vi "DAE Simple Pendulum Simulation_Draw Coord.vi"(3 "picture in":picture) -> (1 "picture out":picture)   [LabVIEW 2023]
doc: "DAE Simple Pendulum Simulation Draw Coordinates"
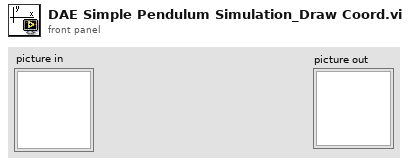
[diagram p1: front panel]
types:
  T1 = cluster{"horizontal":enum16{"left", "center", "right"}, "vertical":enum16{"top", "center", "bottom"}}
  T2 = cluster{"Font Name:":string, "Size":i16, "Strikeout?":bool, "Italic?":bool, "Underline?":bool, "Outline?":bool, "Shadow?":bool, "Bold?":bool}
  T3 = enum16{"User-specified Font", "Application Font", "System Font", "Dialog Font"}
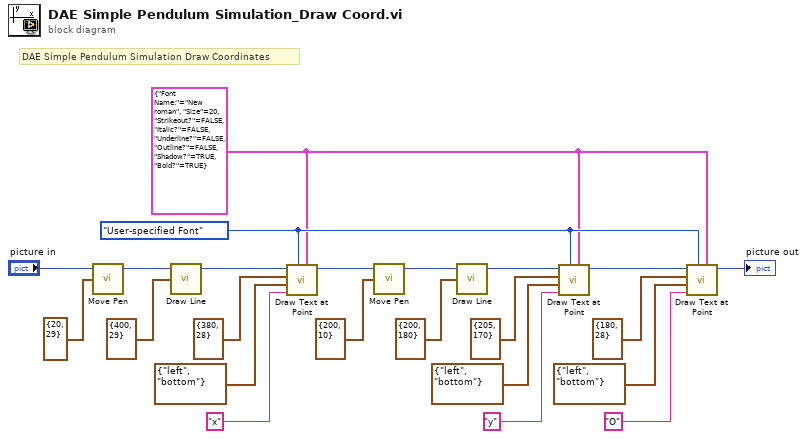
[diagram p0: block diagram]
diagram:
  w21 = T2 {"Font Name:"="New roman", "Size"=20, "Strikeout?"=FALSE, "Italic?"=FALSE, "Underline?"=FALSE, "Outline?"=FALSE, "Shadow?"=TRUE, "Bold?"=TRUE} ("[user-specified font]")
  w22 = T3."User-specified Font" ("desired font(Application)")
  # "DAE Simple Pendulum Simulation Draw Coordinates"
  n1 = call <vilib>:"Move Pen.vi"("new position"=cluster{"x":i16, "y":i16} {"x"=20, "y"=29}, "picture"="picture in") -> ("new picture"=w3:picture)  [unwired: 1 in, 2 out]
  n2 = call <vilib>:"Draw Line.vi"("picture"=w3, "end point"=cluster{"x":i16, "y":i16} {"x"=400, "y"=29}) -> ("new picture"=w5:picture)  [unwired: 3 in, 4 out]
  n3 = call <vilib>:"Draw Text at Point.vi"("[user-specified font]"=w21, "desired font(Application)"=w22, "text"="x", "alignment(left, top)"=T1 {"horizontal"=enum."left", "vertical"=enum."bottom"}, "origin"=cluster{"x":i16, "y":i16} {"x"=380, "y"=28}, "picture"=w5) -> ("new picture"=w9:picture)  [unwired: 3 in, 2 out]
  n4 = call <vilib>:"Move Pen.vi"("new position"=cluster{"x":i16, "y":i16} {"x"=200, "y"=10}, "picture"=w9) -> ("new picture"=w11:picture)  [unwired: 1 in, 2 out]
  n5 = call <vilib>:"Draw Line.vi"("picture"=w11, "end point"=cluster{"x":i16, "y":i16} {"x"=200, "y"=180}) -> ("new picture"=w13:picture)  [unwired: 3 in, 4 out]
  n6 = call <vilib>:"Draw Text at Point.vi"("[user-specified font]"=w21, "desired font(Application)"=w22, "text"="y", "alignment(left, top)"=T1 {"horizontal"=enum."left", "vertical"=enum."bottom"}, "origin"=cluster{"x":i16, "y":i16} {"x"=205, "y"=170}, "picture"=w13) -> ("new picture"=w17:picture)  [unwired: 3 in, 2 out]
  n7 = call <vilib>:"Draw Text at Point.vi"("[user-specified font]"=w21, "desired font(Application)"=w22, "text"="O", "alignment(left, top)"=T1 {"horizontal"=enum."left", "vertical"=enum."bottom"}, "origin"=cluster{"x":i16, "y":i16} {"x"=180, "y"=28}, "picture"=w17) -> ("new picture"=→"picture out":picture)  [unwired: 3 in, 2 out]
